vi "Set One Movable.vi"(10 "Movable in":refnum<class "Game Board Component.lvclass">, 11 "Collision in":refnum<class "Collision.lvclass">) -> (3 "Collision out":refnum<class "Collision.lvclass">)   [LabVIEW 2024, in "Collision.lvclass"]
doc: "MIT Licence\nCopyright (c) 2024 David Grollier"
uses:
  Collision.lvclass
  Game Componants/Game Board Component/Game Board Component.lvclass
  Collision.lvclass/Collision.ctl
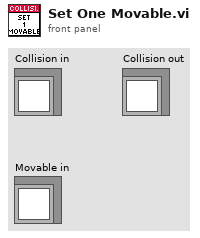
[diagram p1: front panel]
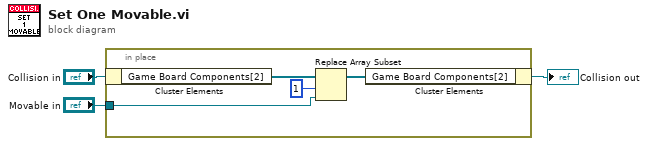
[diagram p0: block diagram]
diagram:
  n1 = in-place {
    in-place-border: "Movable in" -> [w4]
    n2 = in-place-cluster #1("Collision in") -> ("Game Board Components[2]"=w7:refnum<class "Game Board Component.lvclass">[])
    n3 = Replace Array Subset(array=w7, new element=w4, index=1) -> (w5:refnum<class "Game Board Component.lvclass">[])
    n4 = in-place-cluster #1("Game Board Components[2]"=w5) -> (→"Collision out":refnum<class "Collision.lvclass">)
  }
